vi "Calibrate BP Sensor2.vi"(6 "Initialize/Close?":bool, 7 "Calibration Standard":dbl, 8 "Error In (No Error)":errorcluster, 9 "Calibrate":bool=TRUE, 10 "Sensor Address In":string="0", 11 "RS232 Port In":refnum<visa-resource-name>="COM11") -> (0 "Error Out":errorcluster, 1 "Sensor Calibrate Response":bool, 2 "Address Out":string, 3 "RS232 Port Out":refnum<visa-resource-name>, 4 "Calibration Response String":string, 5 "Calibration Response":T1)   [LabVIEW 2016]
doc: "Sends an SDI-12 Send Identification Command, and returns the various attributes from the sensor's response.\n\nThe total size by the sensor must be 22-35 in size (inclusive), or this VI will return an error."
panel:
  out "Command":string
  # "(c) 2008 National Instruments.  ALL RIGHTS RESERVED."
  # "The following are required,\nor are optional, for the sensors\nto respond with:"
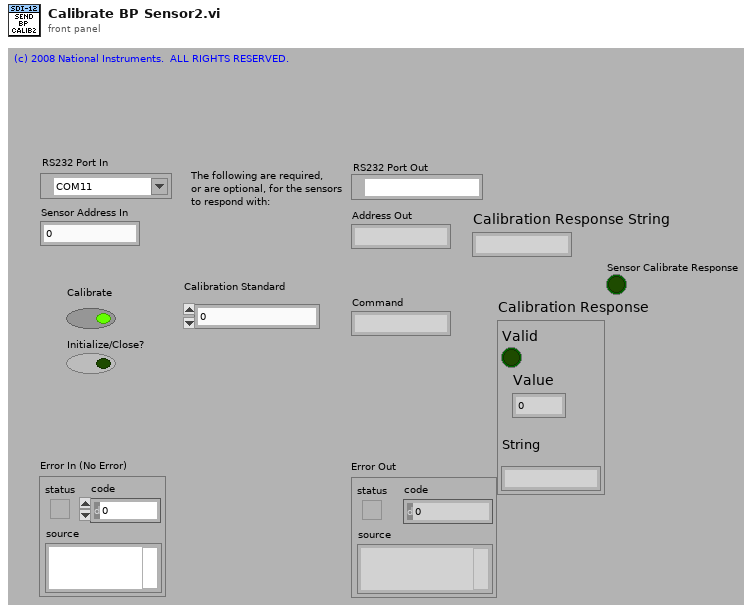
[diagram p1: front panel]
types:
  T1 = cluster{"Valid":bool, "Value":dbl, "\nString ":string}
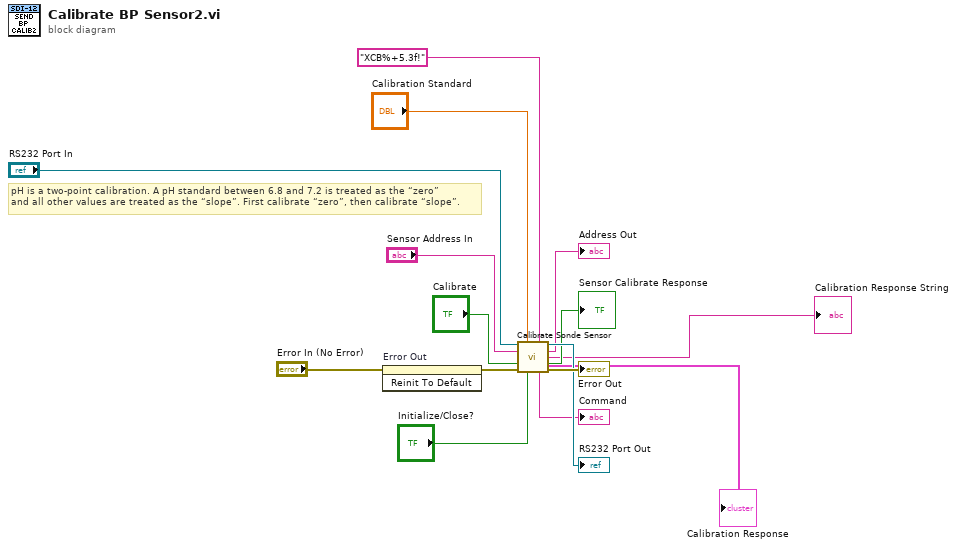
[diagram p0: block diagram]
diagram:
  # "pH is a two-point calibration. A pH standard between 6.8 and 7.2 is treated as the “zero”\nand all other values are treated as the “slope”. First calibrate “zero”, then calibrate “slope”."
  n1 = invoke on="Error Out" class="Clust (strict)" method="Reinit To Default"(error in="Error In (No Error)") -> (error out=w7:errorcluster)  [unwired: 2 in, 2 out]
  n2 = call "Calibrate Sonde Sensor.vi"("RS232 Port In"="RS232 Port In", "Calibration Standard"="Calibration Standard", "Calibrate command  string"="XCB%+5.3f!", "Sensor Address In"="Sensor Address In", "Calibrate"="Calibrate", "Error In (No Error)"=w7, "Initialize/Close?"="Initialize/Close?") -> ("RS232 Port Out"=→"RS232 Port Out":refnum<visa-resource-name>, "Address Out"=→"Address Out":string, "Calibration Response String"=→"Calibration Response String":string, "Sensor Calibrate Response"=→"Sensor Calibrate Response":bool, "Calibration Response"=→"Calibration Response":T1, "Command"=→"Command":string, "Error Out"=→"Error Out":errorcluster)  [unwired: 2 in]
